vi "My2DModel4.vi"(8 "L 2":dbl(slide)=115.0 scale=0.0..200.0, 9 "L 1":dbl(slide)=80.0 scale=0.0..200.0) -> (1 "end effector":cluster{dbl, dbl}={159.01647214211073, 1.9100783062530127} {"?" format="%.1f"; "?" format="%#.1f"}, 3 "2D Picture":picture)   [LabVIEW 2024]
uses:
  Control 1.ctl
panel:
  out "appended array 3":dbl[](array[numeric])
  out "appended array 2":dbl[][](array[numeric])
  out "size(s) 3":i32
  out "size(s) 2":i32
  out "Array":cluster{dbl, dbl}[](array[cluster])
  out "size(s)":i32
  out "appended array":cluster{dbl, dbl}[](array[cluster])
  out "angle":dbl
  out "mag":dbl
  # "A 2"
  # "L2"
  # "L1"
  # "A 1"
  # "mm"
  # "mm"
  # "mm"
  # "mm"
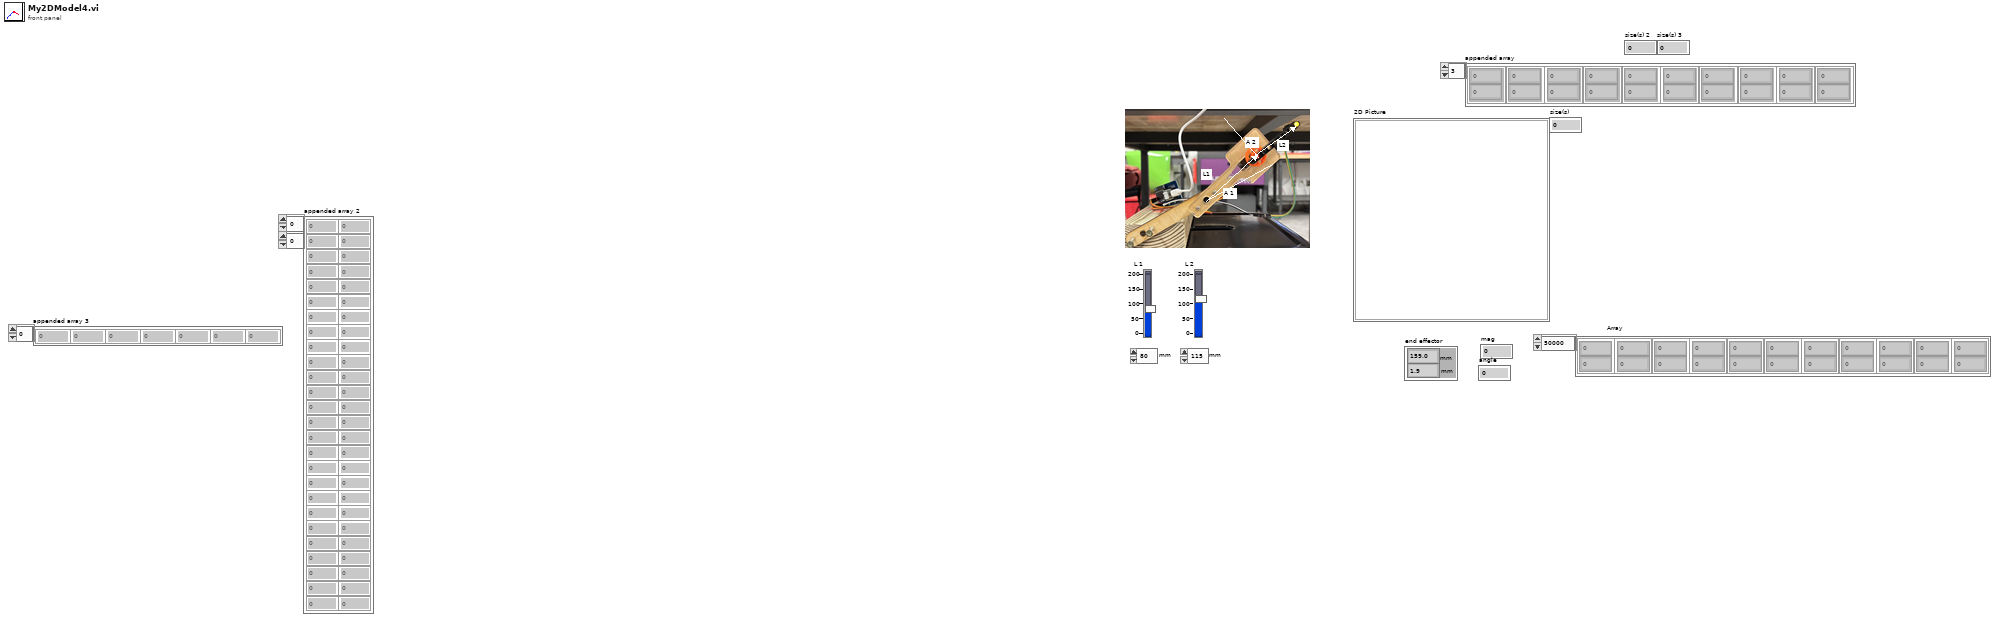
[diagram p1: front panel]
types:
  T1 = typedef "Control 1.ctl" = picture
  T2 = cluster{"Width":u16, "Style":enum32{"Solid", "Dash", "Dot", "DashDot", "DashDotDot"}}
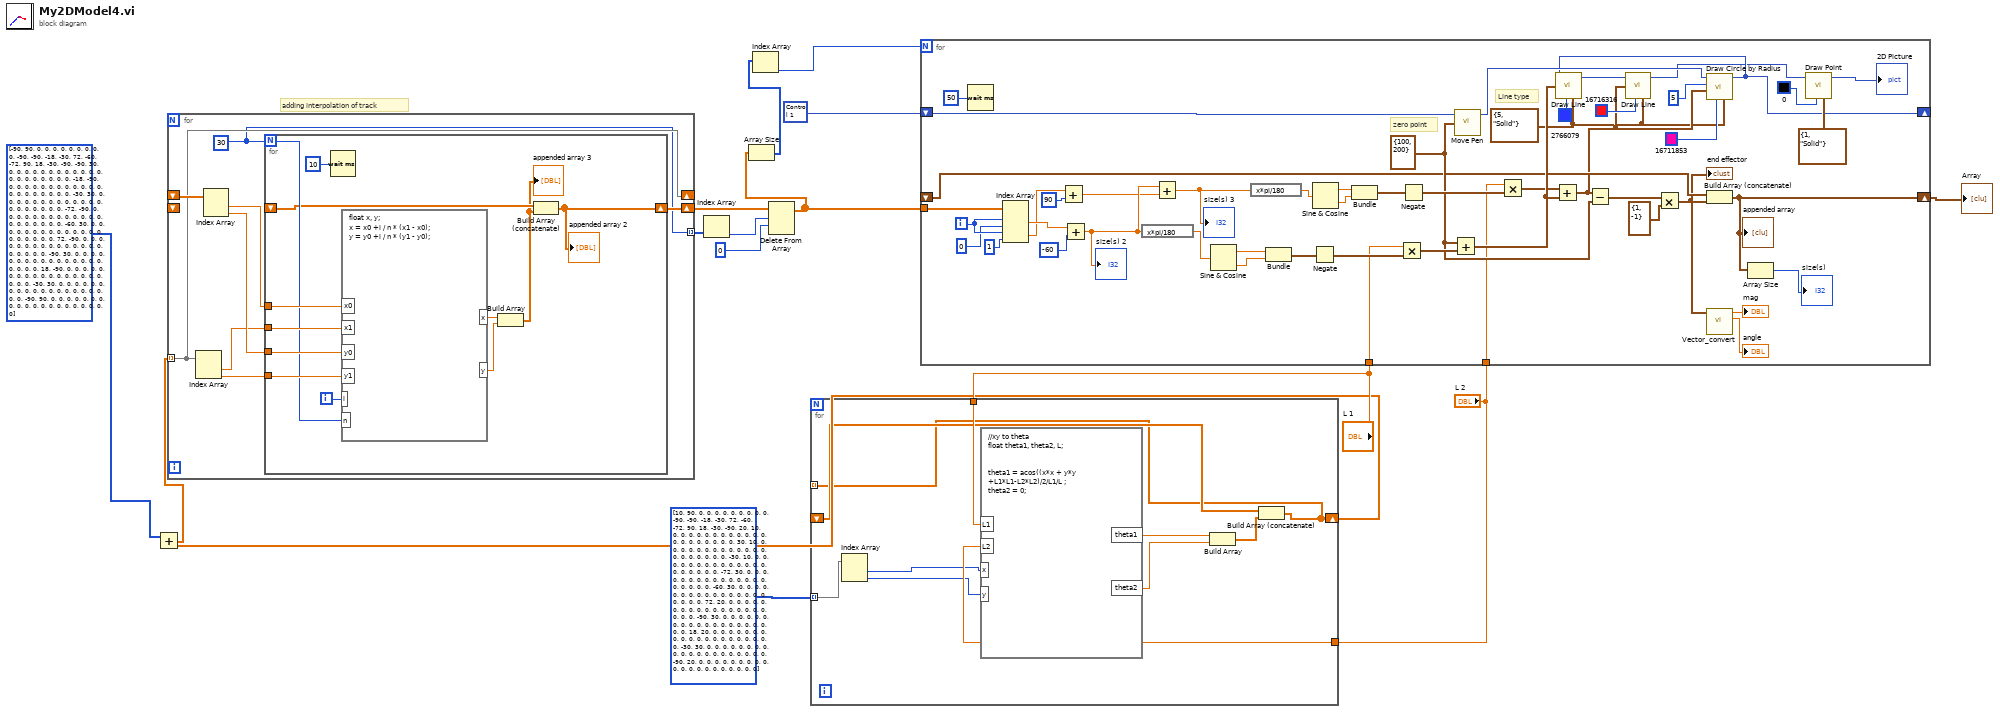
[diagram p0: block diagram]
diagram:
  # "adding interpolation of track"
  n1 = for {
    tunnel: "L 1" -> [w25]
    tunnel: "L 2" -> [w24]
    tunnel: i32[][] [[10, 90, 0, 0, 0, 0, 0, 0, 0, 0, 0, -90, -90, -18, -30, 72, -60, -72, 90, 18, -30, -90], [20, 10, 0, 0, 0, 0, 0, 0, 0, 0, 0, 0, 0, 0, 0, 0, 0, 0, 0, 0, 0, 0], [30, 10, 0, 0, 0, 0, 0, 0, 0, 0, 0, 0, 0, 0, 0, 0, 0, 0, 0, 0, 0, 0], [-30, 10, 0, 0, 0, 0, 0, 0, 0, 0, 0, 0, 0, 0, 0, 0, 0, 0, 0, 0, 0, 0], [-72, 30, 0, 0, 0, 0, 0, 0, 0, 0, 0, 0, 0, 0, 0, 0, 0, 0, 0, 0, 0, 0], [-60, 30, 0, 0, 0, 0, 0, 0, 0, 0, 0, 0, 0, 0, 0, 0, 0, 0, 0, 0, 0, 0], [72, 20, 0, 0, 0, 0, 0, 0, 0, 0, 0, 0, 0, 0, 0, 0, 0, 0, 0, 0, 0, 0], [-90, 30, 0, 0, 0, 0, 0, 0, 0, 0, 0, 0, 0, 0, 0, 0, 0, 0, 0, 0, 0, 0], [18, 20, 0, 0, 0, 0, 0, 0, 0, 0, 0, 0, 0, 0, 0, 0, 0, 0, 0, 0, 0, 0], [-30, 30, 0, 0, 0, 0, 0, 0, 0, 0, 0, 0, 0, 0, 0, 0, 0, 0, 0, 0, 0, 0], [-90, 20, 0, 0, 0, 0, 0, 0, 0, 0, 0, 0, 0, 0, 0, 0, 0, 0, 0, 0, 0, 0]] -> [w23] mode=indexing
    shift-right: [w16] -> w3
    shift-left: _ -> [w17]
    tunnel: [w16] -> _ mode=indexing
    n2 = Index Array(array=w23) -> (element #1=w22:i32, element #2=w21:i32)  [unwired: 2 in]
    n3 = formula code="//xy to theta\nfloat theta1, theta2, L;\n\n\ntheta1 = acos((x*x + y*y +L1*L1-L2*L2)/2/L1/L ;\ntheta2 = 0;"("L1"=w25, "L2"=w24, "x"=w22, "y"=w21) -> ("theta1"=w20:dbl, "theta2"=w19:dbl)
    n4 = Build Array(w20, w19) -> (w18:dbl[])
    n5 = Build Array (concatenate)(w17, w18) -> (w16:dbl[][])
  }
  n6 = Add(x=i32[][] [[-90, 90, 0, 0, 0, 0, 0, 0, 0, 0, 0, -90, -90, -18, -30, 72, -60, -72, 90, 18, -30, -90], [-90, 30, 0, 0, 0, 0, 0, 0, 0, 0, 0, 0, 0, 0, 0, 0, 0, 0, 0, 0, 0, 0], [-18, -90, 0, 0, 0, 0, 0, 0, 0, 0, 0, 0, 0, 0, 0, 0, 0, 0, 0, 0, 0, 0], [-30, 30, 0, 0, 0, 0, 0, 0, 0, 0, 0, 0, 0, 0, 0, 0, 0, 0, 0, 0, 0, 0], [-72, -90, 0, 0, 0, 0, 0, 0, 0, 0, 0, 0, 0, 0, 0, 0, 0, 0, 0, 0, 0, 0], [-60, 30, 0, 0, 0, 0, 0, 0, 0, 0, 0, 0, 0, 0, 0, 0, 0, 0, 0, 0, 0, 0], [72, -90, 0, 0, 0, 0, 0, 0, 0, 0, 0, 0, 0, 0, 0, 0, 0, 0, 0, 0, 0, 0], [-90, 30, 0, 0, 0, 0, 0, 0, 0, 0, 0, 0, 0, 0, 0, 0, 0, 0, 0, 0, 0, 0], [18, -90, 0, 0, 0, 0, 0, 0, 0, 0, 0, 0, 0, 0, 0, 0, 0, 0, 0, 0, 0, 0], [-30, 30, 0, 0, 0, 0, 0, 0, 0, 0, 0, 0, 0, 0, 0, 0, 0, 0, 0, 0, 0, 0], [-90, 90, 0, 0, 0, 0, 0, 0, 0, 0, 0, 0, 0, 0, 0, 0, 0, 0, 0, 0, 0, 0]], y=w3) -> (x+y=w1:dbl[][])
  n7 = for {
    tunnel: w1 -> [w28] mode=indexing
    shift-right: [w27] -> w13
    shift-left: _ -> [_]
    shift-right: [w28] -> _
    shift-left: _ -> [w32]
    tunnel: [w26] -> w12 mode=indexing
    w26 = 30
    n8 = Index Array(array=w28) -> (element #1=w30:dbl, element #2=w29:dbl)  [unwired: 2 in]
    n9 = Index Array(array=w32) -> (element #1=w33:dbl, element #2=w31:dbl)  [unwired: 2 in]
    n10 = for {
      N: w26 -> [w40]
      tunnel: w33 -> [w45]
      tunnel: w31 -> [w44]
      tunnel: w29 -> [w43]
      tunnel: w30 -> [w42]
      shift-right: [w34] -> w27
      shift-left: _ -> [w36]
      i -> [w41]
      n11 = Wait (ms)(milliseconds to wait=10) -> ()  [unwired: 1 out]
      n12 = formula code="float x, y;\nx = x0 +i / n * (x1 - x0);\ny = y0 +i / n * (y1 - y0);"("x0"=w45, "x1"=w42, "y0"=w44, "y1"=w43, "i"=w41, "n"=w40) -> ("x"=w38:dbl, "y"=w39:dbl)
      n13 = Build Array(w38, w39) -> (w35:dbl[])
      "appended array 3" <- w35
      n14 = Build Array (concatenate)(w36, w35) -> (w34:dbl[][])
      "appended array 2" <- w34
    }
  }
  n15 = Index Array(array=w12) -> (element=w11:i32)  [unwired: 1 in]
  n16 = Delete From Array(array=w13, length=w11, index (row)=u32 0 ("milliseconds to wait")) -> (array with subset deleted=w9:dbl[][])  [unwired: 1 in, 1 out]
  n17 = Array Size(array=w9) -> (size(s)=w8:i32[])
  n18 = Index Array(array=w8) -> (element=w7:i32)  [unwired: 1 in]
  n19 = for {
    N: w7 -> [_]
    shift-right: [w69] -> w15
    shift-left: _ -> [w71]
    shift-right: [w49] -> _
    shift-left: T1 data[5B] ("new picture") -> [w60]
    tunnel: w9 -> [w66]
    tunnel: "L 1" -> [w47]
    tunnel: "L 2" -> [w46]
    i -> [w63]
    w53 = T2 {"Width"=5, "Style"=enum."Solid"} ("pen")
    w76 = cluster{"x":i16, "y":i16} {"x"=100, "y"=200} ("new position")
    # "zero point"
    # "Line type"
    n20 = Wait (ms)(milliseconds to wait=u32 50) -> ()  [unwired: 1 out]
    n21 = Index Array(array=w66, index (row) #1=w63, index (col) #1=i16 0 ("x"), index (row) #2=w63, index (col) #2=i16 1 ("x")) -> (element #1=w65:dbl, element #2=w64:dbl)
    n22 = Add(x=w64, y=i16 90 ("x")) -> (x+y=w57:dbl)
    n23 = Add(x=w65, y=i16 -60 ("x")) -> (x+y=w58:dbl)
    "size(s) 2" <- w58
    n24 = expression code="x*pi/180"(w58) -> (w80:dbl)
    n25 = Add(x=w58, y=w57) -> (x+y=w56:dbl)
    "size(s) 3" <- w56
    n26 = Sine & Cosine(0:w80) -> (1:w88:dbl, 2:w89:dbl)
    n27 = expression code="x*pi/180"(w56) -> (w84:dbl)
    n28 = Bundle(w88, w89) -> (w81:cluster{dbl, dbl})  [unwired: 1 in]
    n29 = Negate(x=w81) -> (-x=w90:cluster{dbl, dbl})
    n30 = Sine & Cosine(0:w84) -> (1:w91:dbl, 2:w92:dbl)
    n31 = Bundle(w91, w92) -> (w83:cluster{dbl, dbl})  [unwired: 1 in]
    n32 = Multiply(x=w47, y=w90) -> (x*y=w82:cluster{dbl, dbl})
    n33 = Negate(x=w83) -> (-x=w93:cluster{dbl, dbl})
    n34 = Add(x=w76, y=w82) -> (x+y=w86:cluster{dbl, dbl})
    n35 = call <vilib>:"Move Pen.vi"("new position"=w76, "picture"=w60) -> ("new picture"=w51:picture)  [unwired: 3 in]
    n36 = Multiply(x=w46, y=w93) -> (x*y=w85:cluster{dbl, dbl})
    n37 = Add(x=w85, y=w86) -> (x+y=w55:cluster{dbl, dbl})
    n38 = Subtract(x=w55, y=w76) -> (x-y=w87:cluster{dbl, dbl})
    n39 = Multiply(x=w87, y=cluster{"x":i16, "y":i16} {"x"=1, "y"=-1} ("new position")) -> (x*y=w70:cluster{dbl, dbl})
    "end effector" <- w70
    n40 = call <vilib>:"Draw Circle by Radius.vi"("pen"=w53, "color(black)"=u32 16711853, "pixel center"=w55, "radius"=u16 5 ("Width"), "picture"=w51) -> ("new picture"=w49:picture)  [unwired: 6 in]
    n41 = call <vilib>:"Draw Line.vi"("picture"=w49, "end point"=w86, "color(black)"=u32 2766079, "pen"=w53) -> ("new picture"=w50:picture)  [unwired: 5 in]
    n42 = call <vilib>:"Draw Line.vi"("picture"=w50, "end point"=w55, "color(black)"=u32 16716316, "pen"=w53) -> ("new picture"=w48:picture)  [unwired: 5 in]
    n43 = Build Array (concatenate)(w71, w70) -> (w69:cluster{dbl, dbl}[])
    "appended array" <- w69
    n44 = call "Vector_convert.vi"("x,y"=w70) -> ("angle"=→"angle":dbl, "mag"=→"mag":dbl)  [unwired: 9 in]
    n45 = Array Size(array=w69) -> (size(s)=→"size(s)":i32)
    n46 = call <vilib>:"Draw Point.vi"("picture"=w48, "color(black)"=u32 0, "pen"=T2 {"Width"=1, "Style"=enum."Solid"}) -> ("new picture"=→"2D Picture":picture)  [unwired: 6 in]
  }
  "Array" <- w15
